vi "Lookup Devices by GUID.vi"(8 "error in (no error)":errorcluster, 10 "GUID":string, 11 "Controller in":refnum<class "Controller.lvclass">) -> (0 "error out":errorcluster, 2 "Dev Obj out":refnum<class "Hardware.lvclass">, 3 "Controller out":refnum<class "Controller.lvclass">)   [LabVIEW 2016, in "Controller Actor.lvlib" / "Controller.lvclass"]
uses:
  <userlib>/Common Components/Controller/Controller.lvclass
  <userlib>/Common Components/Hardware/Abstract Hardware/Hardware.lvclass
  <userlib>/Common Components/Controller/Controller.lvclass/Controller.ctl
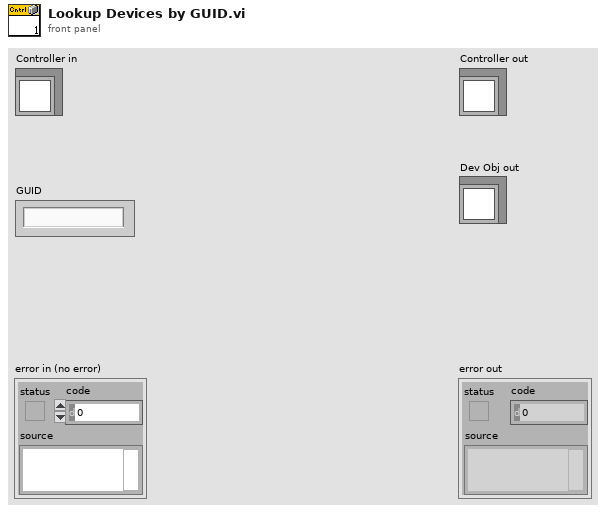
[diagram p1: front panel]
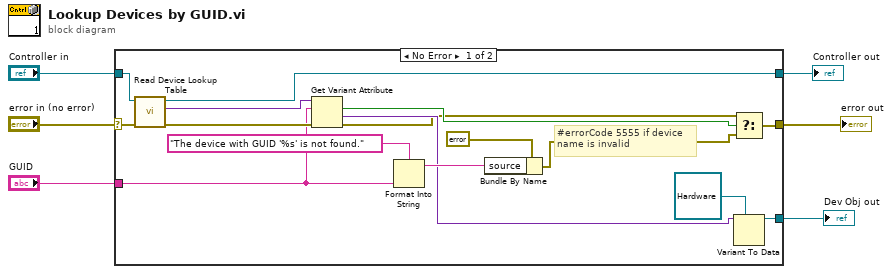
[diagram p0: block diagram]
diagram:
  n1 = case shown="No Error" "error in (no error)" {
    selector: "error in (no error)" -> [w18 w24]
    tunnel: [w10 w24] -> w5
    tunnel: [w20 w23] -> w3
    tunnel: "Controller in" -> [w22 w23]
    tunnel: "GUID" -> [w8 _]
    tunnel: [w7 _] -> w1
    frame No Error {
      # "#errorCode 5555 if device\nname is invalid"
      n2 = call <userlib>:"Read Device Lookup Table.vi"("error in (no error)"=w18, "Controller in"=w22) -> ("error out"=w19:errorcluster, "Device Lookup Table (Device GUID -> Device Object)"=w21:variant, "Controller out"=w20:refnum<class "Controller.lvclass">)  [unwired: 7 in]
      n3 = Get Variant Attribute(Variant=w21, name=w8, error in=w19) -> (found=w11:bool, value=w12:variant, error out=w9:errorcluster)  [unwired: 1 in, 1 out]
      n4 = Format Into String(format string="The device with GUID '%s' is not found." ("source"), w8) -> (resulting string=w15:string)  [unwired: 2 in, 1 out]
      n5 = Bundle By Name(cluster=errorcluster {"status"=TRUE, "code"=5555, "source"="Device '%s' Invalid"} ("error constant"), "source"=w15) -> (w13:errorcluster)
      n6 = Select(t=w9, s=w11, f=w13) -> (s? t:f=w10:errorcluster)
      n7 = Variant To Data(type=refnum<class "Hardware.lvclass"> refnum ("Hardware.lvclass"), Variant=w12) -> (data=w7:refnum<class "Hardware.lvclass">)  [unwired: 1 in, 1 out]
    }
    frame Error {
    }
  }
  "error out" <- w5
  "Controller out" <- w3
  "Dev Obj out" <- w1
